vi "Write Worktable.vi"(8 "error in":errorcluster, 10 "WorkTable in":refnum<class "WorkTable Class.lvclass">=refnum, 11 "Potting Procedure in":refnum<class "Potting Procedure.lvclass">) -> (0 "error out":errorcluster, 3 "Potting Procedure out":refnum<class "Potting Procedure.lvclass">)   [LabVIEW 2017, in "Potting Procedure.lvclass"]
uses:
  Potting Procedure.lvclass
  Shared Components/Gantry Class/Gantry Class.lvclass
  Shared Components/FlexWorktable/FlexWorktable.lvclass
  Shared Components/WorkTable Class/WorkTable Class.lvclass
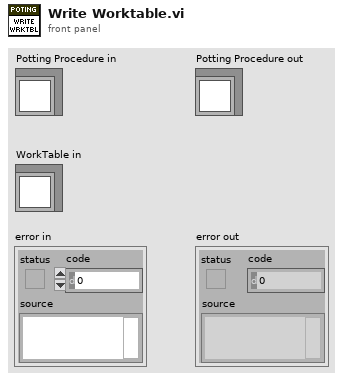
[diagram p1: front panel]
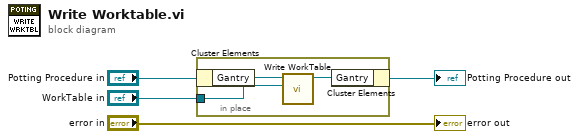
[diagram p0: block diagram]
diagram:
  n1 = in-place {
    in-place-border: "WorkTable in" -> [w7]
    n2 = in-place-cluster #1("Potting Procedure in") -> ("Gantry"=w6:refnum<class "Gantry Class.lvclass">)
    n3 = call-dynamic "Write WorkTable.vi"("FlexWorktable"=w7, "Gantry Class in"=w6) -> ("Gantry Class out"=w5:refnum<class "Gantry Class.lvclass">)  [unwired: 8 in, 1 out]
    n4 = in-place-cluster #1("Gantry"=w5) -> (→"Potting Procedure out":refnum<class "Potting Procedure.lvclass">)
  }
  "error out" <- "error in"
